vi "ResearcgStandingFrame-V2.1.vi"() -> ()   [LabVIEW 2012]
doc: "Use this template to build a simple state machine design pattern. Each state executes code and determines which state to transition to."
uses:
  controls/State.ctl
  <vilib>/DAQmx/read.llb/DAQmx Read (Analog 2D DBL NChan NSamp).vi
  <vilib>/DAQmx/create/channels.llb/DAQmx Create Channel (AI-Voltage-Basic).vi
  <vilib>/DAQmx/configure/timing.llb/DAQmx Timing (Sample Clock).vi
  <vilib>/DAQmx/create/channels.llb/DAQmx Create Channel (CO-Pulse Generation-Frequency).vi
  <vilib>/DAQmx/configure/timing.llb/DAQmx Timing (Implicit).vi
  <vilib>/DAQmx/miscellaneous.llb/DAQmx Fill In Error Info.vi
  <vilib>/Utility/file.llb/Write To Spreadsheet File (DBL).vi
panel:
  out "refnum out":refnum<file>
  in  "Tab Control":T1(tab)
  in  "?":bool
  out "Center Mass Left Force Plate":cluster{dbl[], dbl[]}(graph)={[-7.494780644696312], [-1.1979086821741642]}
  in  "Save":bool
  in  "stop":bool
  out "Newton Force Readings File Path":path=path "C:/Documents and Settings/z00323/My Documents/Standing Frame/test data/StandingFrameTEST39.dat"
  in  "Newtons":bool
  out "Voltage Readings File Path":path=path "C:/Documents and Settings/z00323/My Documents/Standing Frame/test data/StandingFrameTEST39.dat"
  out "R-FP-Z":dbl
  out "R-FP-Y":dbl
  out "R-FP-X":dbl
  out "R-LC-Z":dbl
  out "R-LC-Y":dbl
  out "R-LC-X":dbl
  out "L-LC-Z":dbl
  out "L-LC-Y":dbl
  out "L-LC-X":dbl
  out "L-FP-X":dbl
  out "L-FP-Y":dbl
  out "L-FP-Z":dbl
  out "String":string caption="Display Unit"
  out "Left Force Plate Z":dbl(slide)=0.43558763460600747 scale=0.0..250.0
  out "Right Force Plate Z":dbl(slide)=0.868584773555102 scale=0.0..250.0
  out "Center Mass Right Force Plate":cluster{dbl[], dbl[]}(graph)
  out "Right Load Cell":cluster{dbl[], dbl[]}(graph)={[0.0, -0.0006862149399022939, 0.0, 0.0], [0.0, 0.005798023167495851, 0.0, 0.0]}
  out "Right Load Cell Z":dbl(slide)=-0.000301685706272135 scale=-50.0..250.0
  out "Left Load Cell Z":dbl(slide)=-0.004073381073294343 scale=-50.0..250.0
  out "Left Load Cell":cluster{dbl[], dbl[]}(graph)={[0.0, -0.0004854170425343219, 0.0, 0.0], [0.0, -0.002818533162237429, 0.0, 0.0]}
  out "Amplitude Unit":string
  out "Right Force PLate Z":dbl(graph)
  out "Left Force Plate Z":dbl(graph)
  out "Right Load Cell Z":dbl(graph)
  out "Right Load Cell Y":dbl(graph)
  out "Right Load Cell X":dbl(graph)
  out "Left Load Cell Z":dbl(graph)
  out "Left Load Cell Y":dbl(graph)
  out "Left Load Cell X":dbl(graph)
  out "Amplitude Unit":string
  out "Loading- Clibration File Path":path
  in  "Save Calibration Results":bool
  in  "Load Previous Calibration Results":bool
  out "Saving- Clibration File Path":path
  out "Baseline Out":dbl[](array[numeric])
  out "Voltages":dbl[](array[numeric])
  in  "New Calibration":bool
  # "FP4"
  # "FP3"
  # "Left Load Cell X\n\nLeft Load Cell Y\n\nLeft Load Cell Z\n\nRight Load Cell X\n\nRight Load Cell Y\n\nRight Load Cell Z"
  # "DAQ Board Connections"
  # "Left Force Plate X1\n\nLeft Force Plate X2\n\nLeft Force Plate Y1\n\nLeft Force Plate Y2\n\nLeft Force Plate Z1\n\nLeft Force Plate Z2\n\nLeft Force Plate Z3\n\nLeft Force Plate Z4"
  # "LX\nLY\nLZ\nRX\nRY\nRZ\nLFX12\nLFX34\nLFY14\nLFY23\nLFZ1\nLFZ2\nLFZ3\nLFZ4\nRFX12\nRFX34\nRFY14\nRFY23\nRFZ1\nRFZ2\nRFZ3\nRFZ4"
  # "32\n33\n34\n35\n36\n37\n0\n1\n2\n3\n4\n5\n6\n7\n16\n17\n18\n19\n20\n21\n22\n23"
  # "Right Force Plate X1\n\nRight Force Plate X2\n\nRight Force Plate Y1\n\nRight Force Plate Y2\n\nRight Force Plate Z1\n\nRight Force Plate Z2\n\nRight Force Plate Z3\n\nRight Force Plate Z4"
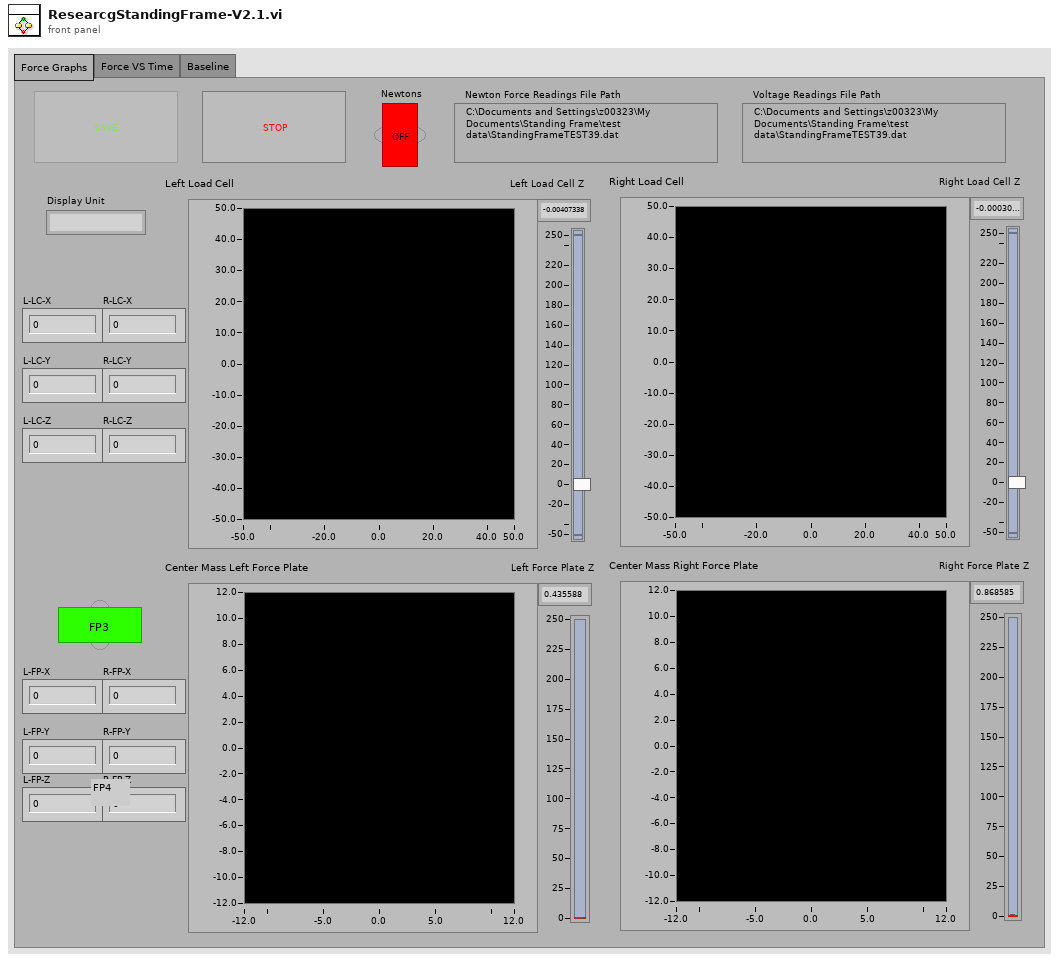
[diagram p1: front panel]
types:
  T1 = enum32{"Force Graphs", "Force VS Time", "Baseline"}
  T2 = typedef "State.ctl" = enum16{"Initialize", "Save", "Main", "Stop"}
  T3 = enum16{"open", "replace", "create", "open or create", "replace or create", "replace or create with confirmation"}
  T4 = enum8{"Enabled", "Disabled", "Disabled and Grayed Out"}
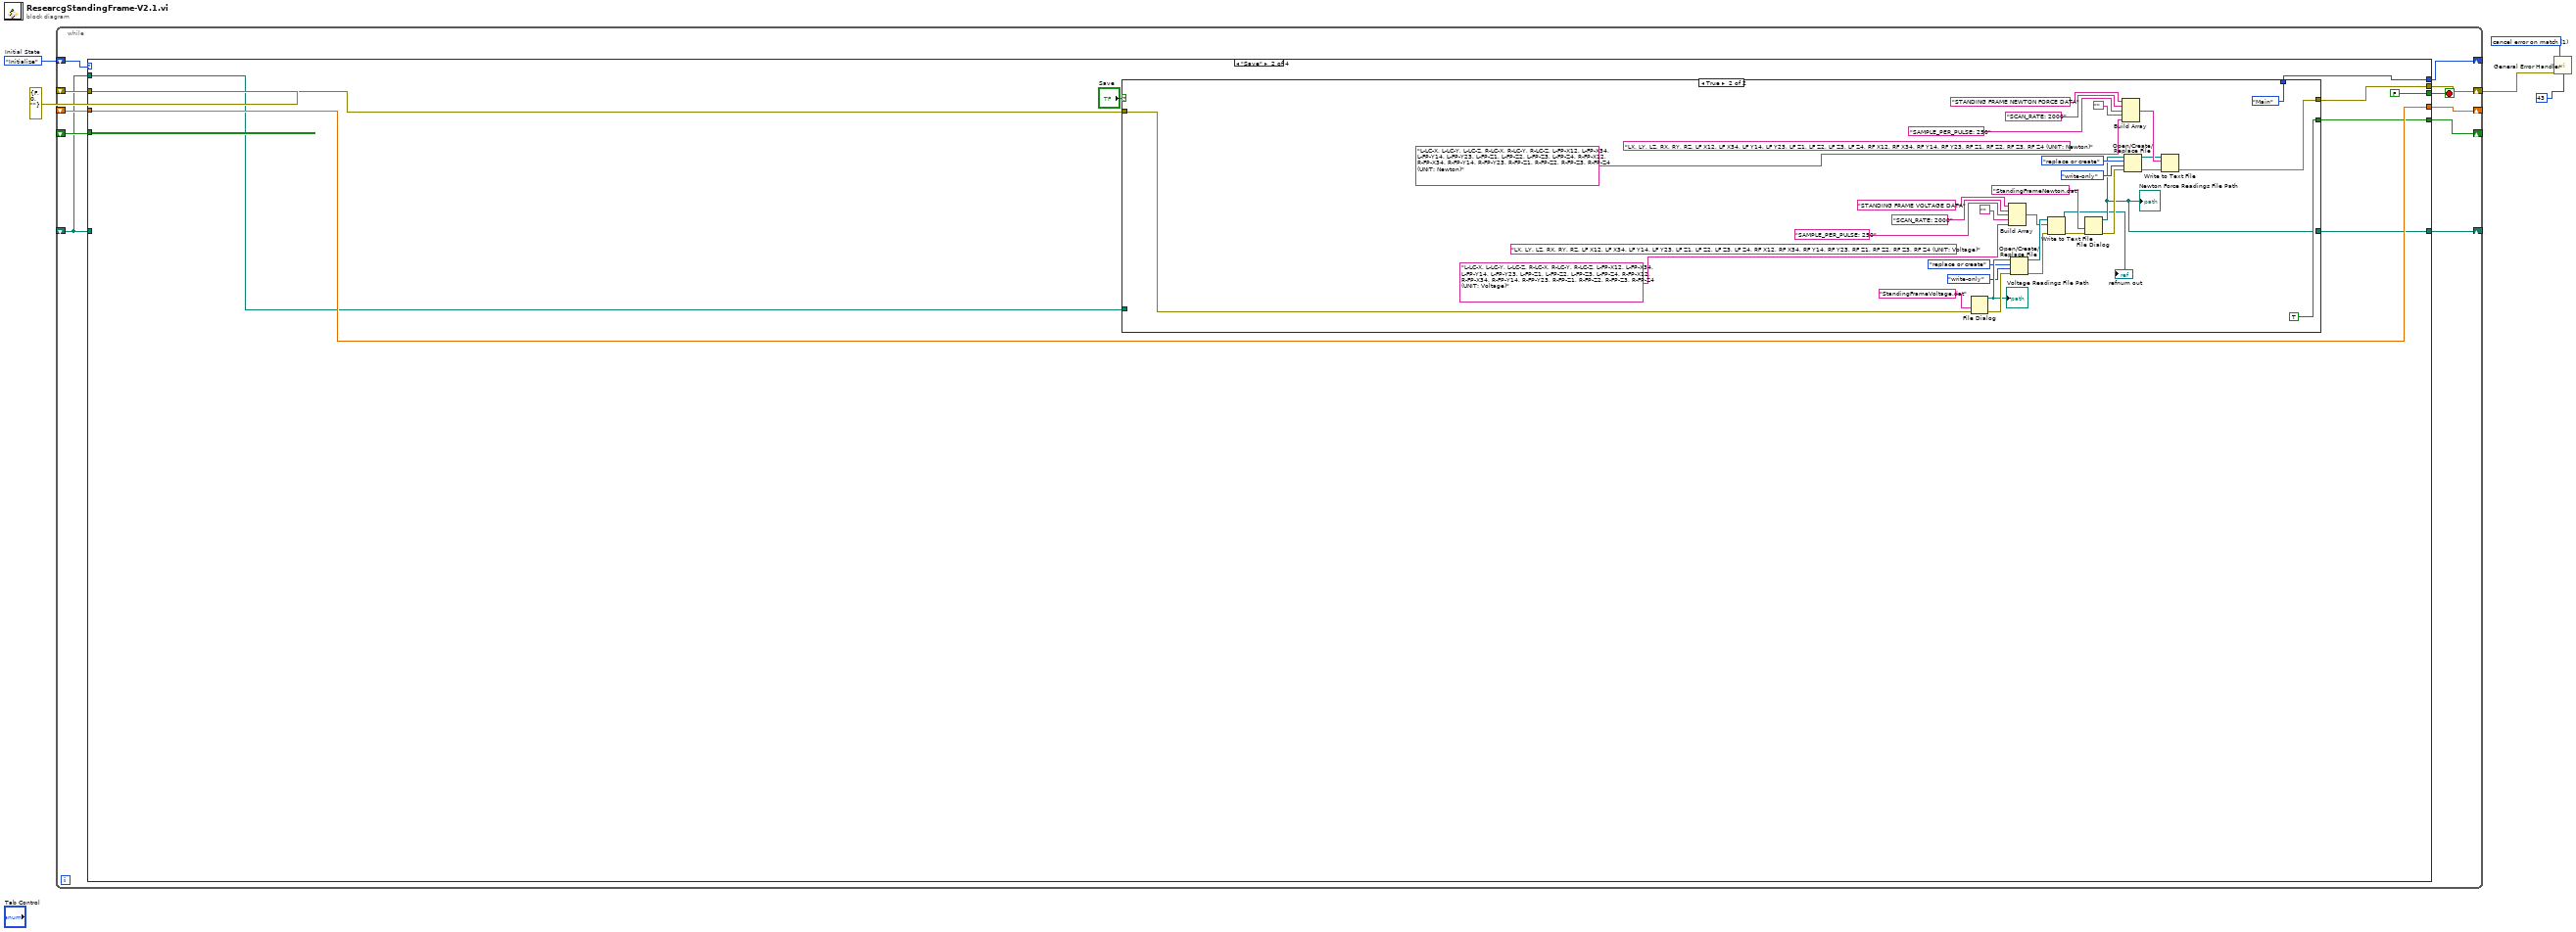
[diagram p0: block diagram]
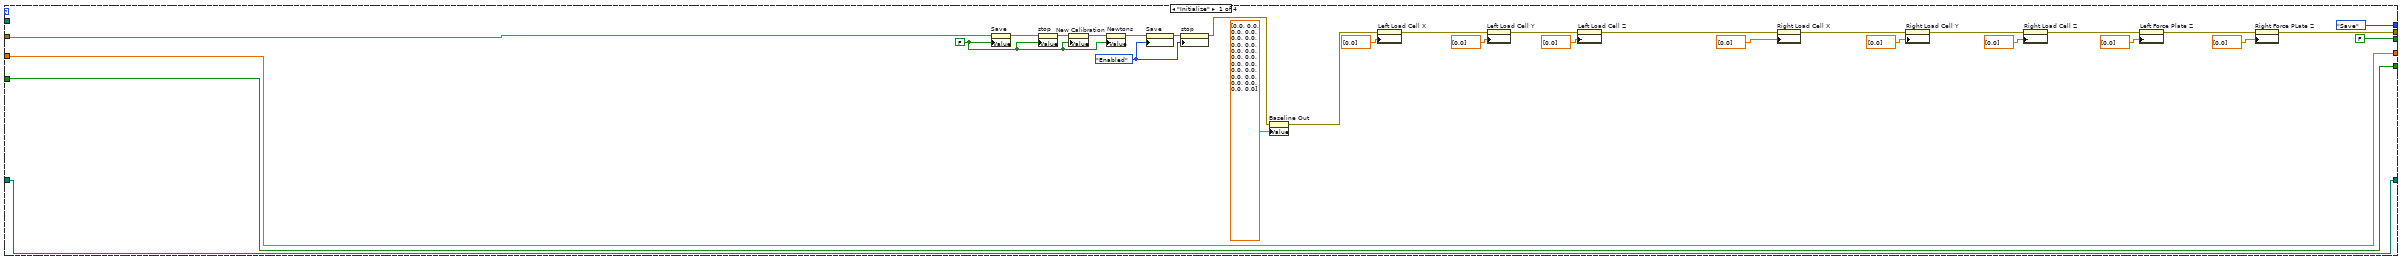
[diagram p2: hidden frame]
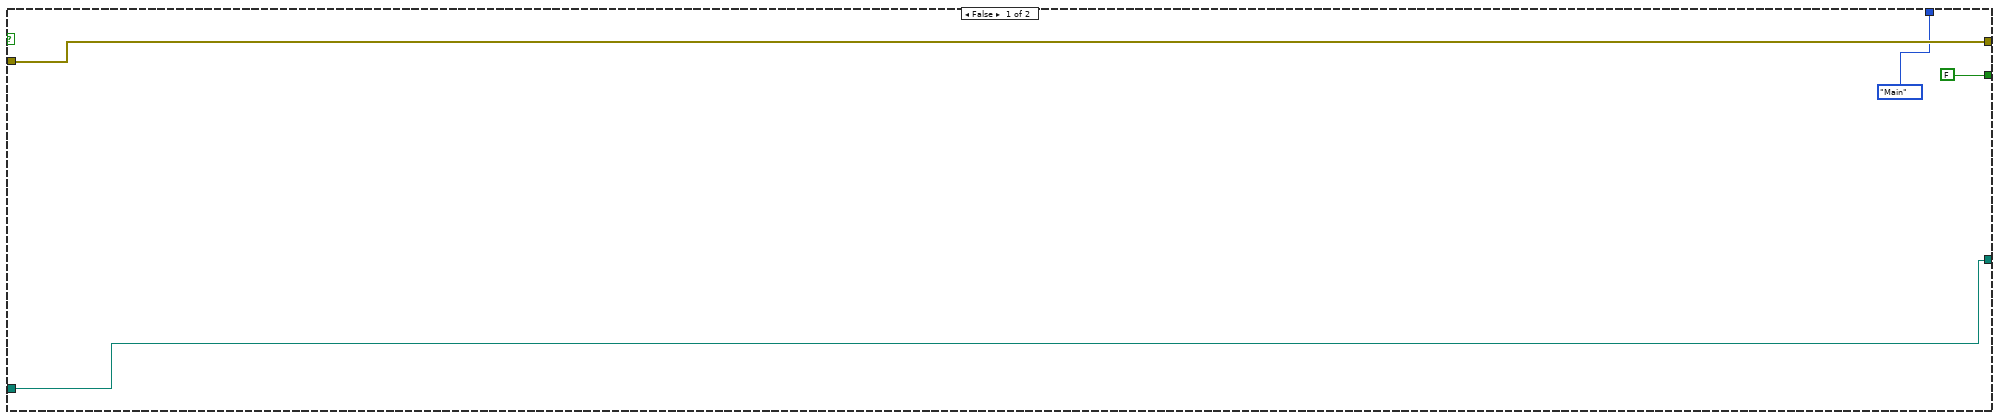
[diagram p3: hidden frame]
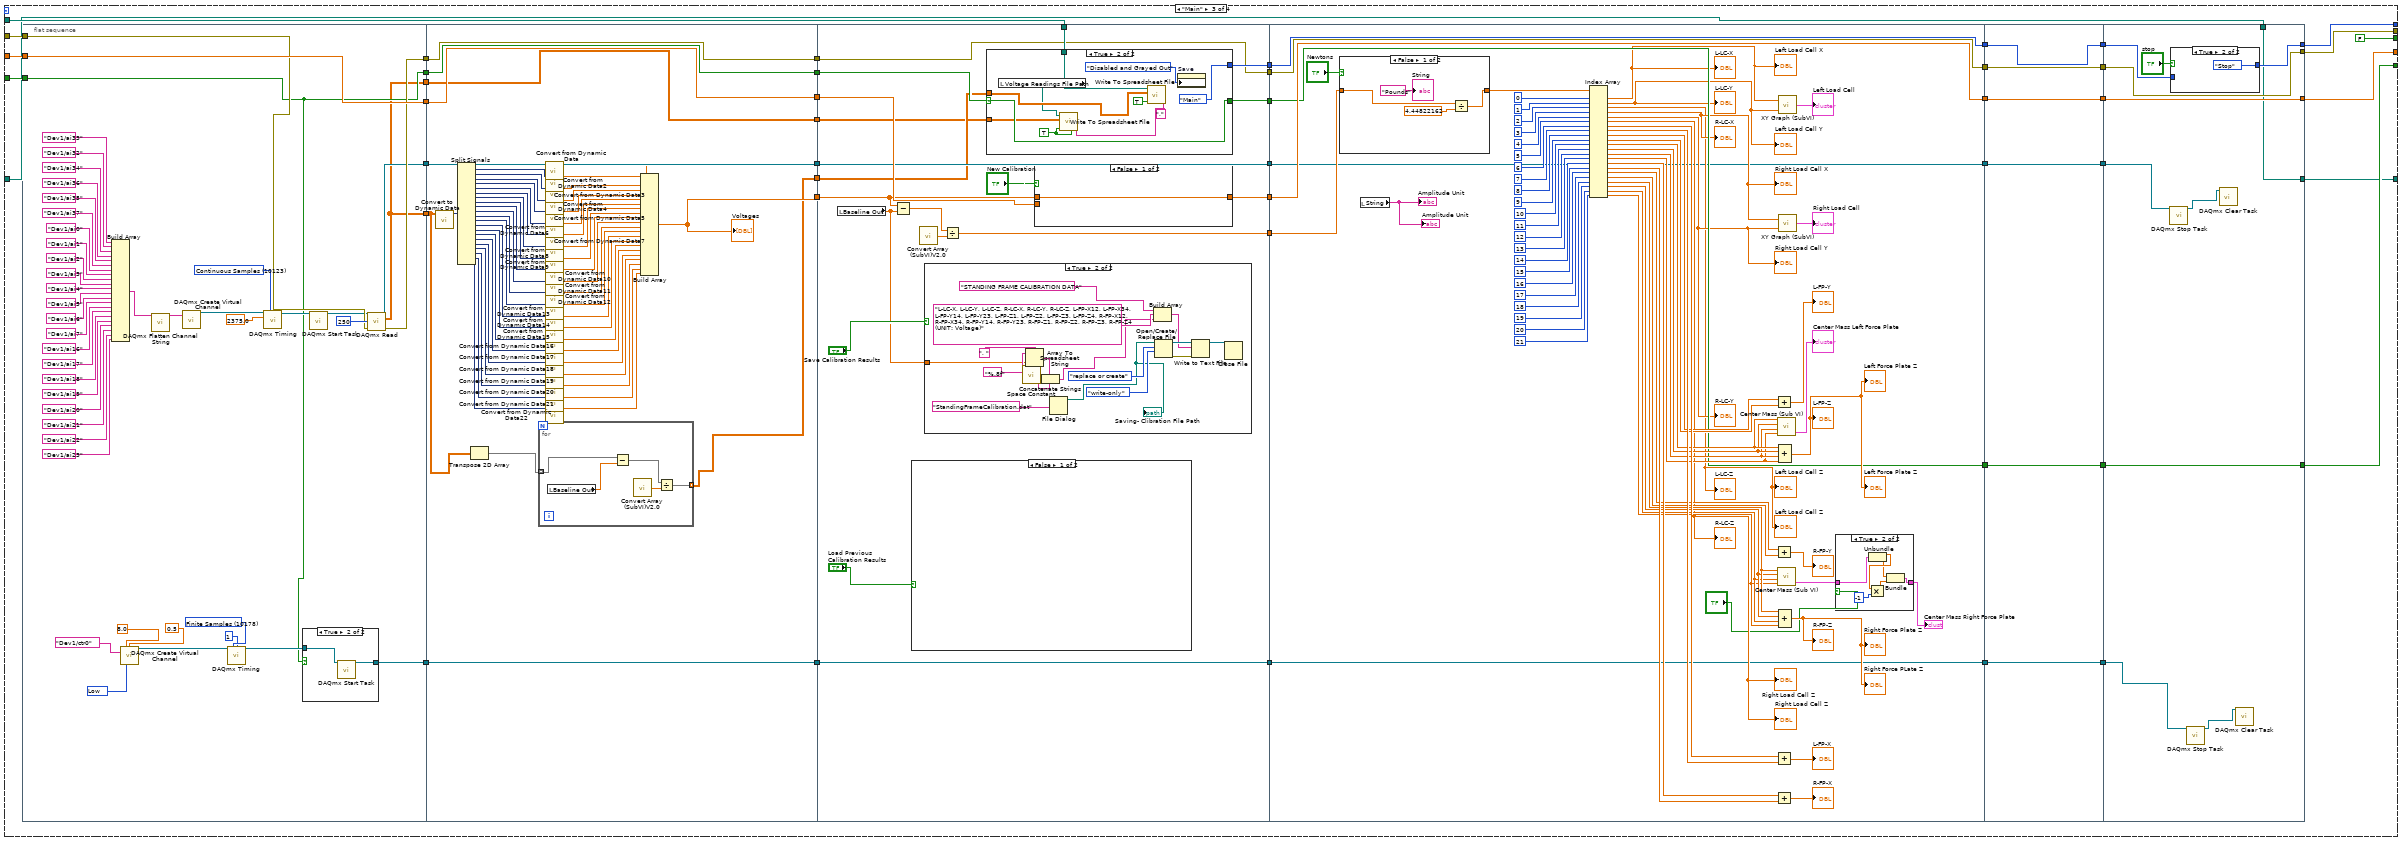
[diagram p4: hidden frame]
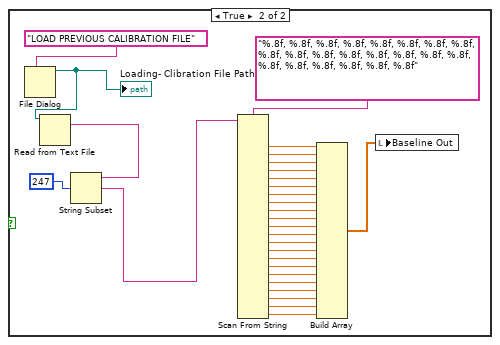
[diagram p6: hidden frame]
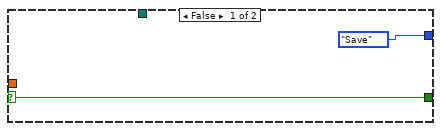
[diagram p8: hidden frame]
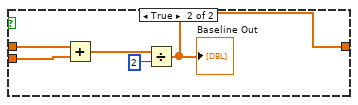
[diagram p9: hidden frame]
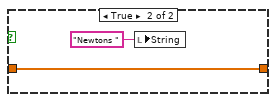
[diagram p11: hidden frame]
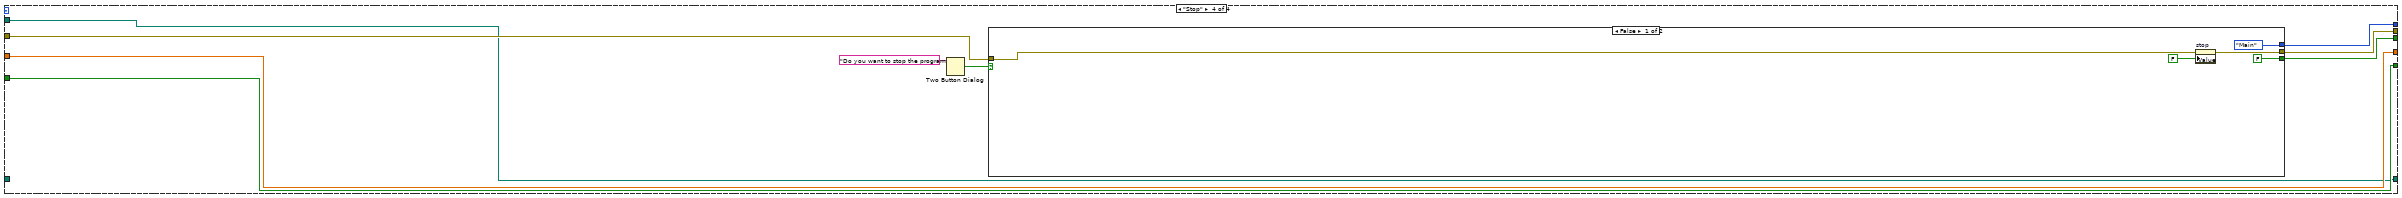
[diagram p13: hidden frame]
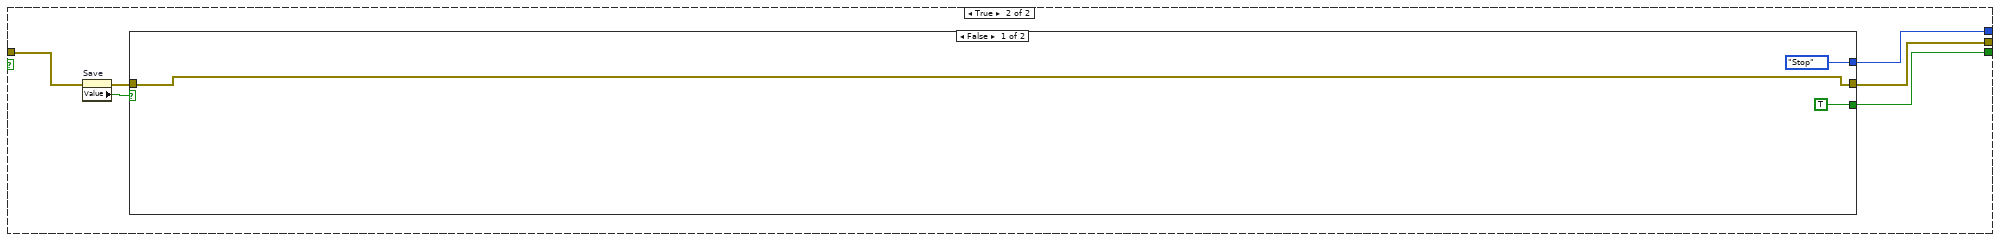
[diagram p14: hidden frame]
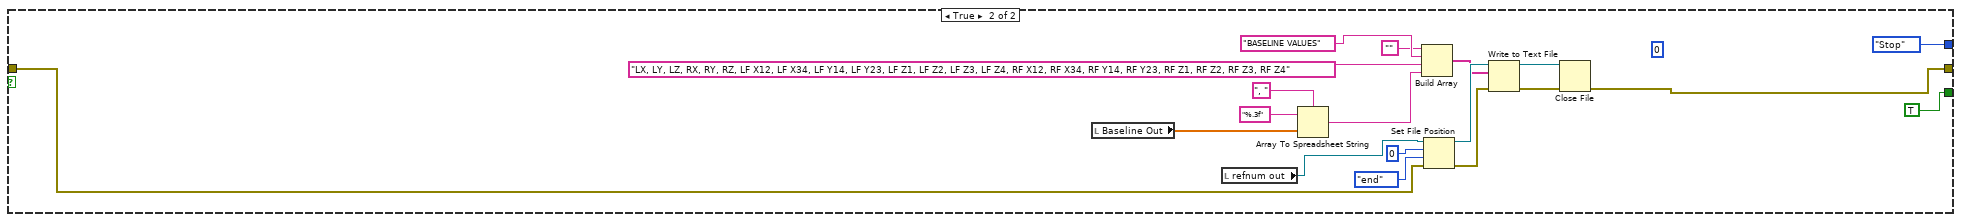
[diagram p15: hidden frame]
diagram:
  w1 = 1 items=["no exception", "cancel error on match", "set error on match"] ("[exception action] (none:0)")
  w5 = State."Initialize"  # Initial State
  n1 = while {
    shift-right: [w16] -> _
    shift-left: w5 -> [w6]
    shift-right: [w13] -> w3
    shift-left: errorcluster {"status"=FALSE, "code"=0, "source"=""} ("error out") -> [w15]
    shift-right: [w11] -> _
    shift-left: _ -> [w12]
    shift-right: [w10] -> _
    shift-left: _ -> [w9]
    shift-right: [w8] -> _
    shift-left: _ -> [w7]
    stop <- w14 stop-if-true
    n2 = case shown="\"Save\"" w6 {
      tunnel: [State."Save" ("Next State") w51 w137 w433] -> w16
      tunnel: [FALSE ("T button?") FALSE FALSE ("T button?") w432] -> w14
      tunnel: w15 -> [w43 w56 w138 w431]
      tunnel: [w20 w55 w127 w430] -> w13
      tunnel: w12 -> [w42 w53 w125 w429]
      tunnel: [w42 w53 w121 w429] -> w11
      tunnel: [w18 w52 w118 w428] -> w10
      tunnel: w9 -> [w18 _ w119 w428]
      tunnel: [w17 w50 w94 w427] -> w8
      tunnel: w7 -> [_ w49 w96 w427]
      tunnel: w7 -> [w17 _ w95 _]
      frame "Initialize" {
        w37 = FALSE ("Begin")
        w46 = T4."Enabled" ("Disabled")
        n3 = property on="Save" class="Bool (strict)"(error in=w43, "Value"=w37) -> (error out=w45:errorcluster)  [unwired: 1 in, 1 out]
        n4 = property on="stop" class="Bool (strict)"(error in=w45, "Value"=w37) -> (error out=w41:errorcluster)  [unwired: 1 in, 1 out]
        n5 = property on="New Calibration" class="Bool (strict)"(error in=w41, "Value"=w37) -> (error out=w39:errorcluster)  [unwired: 1 in, 1 out]
        n6 = property on="Newtons" class="Bool (strict)"(error in=w39, "Value"=w37) -> (error out=w38:errorcluster)  [unwired: 1 in, 1 out]
        n7 = property on="Save" class="Bool (strict)"(error in=w38, "DisabledEnum"=w46) -> (error out=w44:errorcluster)  [unwired: 1 in, 1 out]
        n8 = property on="stop" class="Bool (strict)"(error in=w44, "DisabledEnum"=w46) -> (error out=w19:errorcluster)  [unwired: 1 in, 1 out]
        n9 = property on="Baseline Out" class="Arr (strict)"(error in=w19, "Value"=dbl[] [0.0, 0.0, 0.0, 0.0, 0.0, 0.0, 0.0, 0.0, 0.0, 0.0, 0.0, 0.0, 0.0, 0.0, 0.0, 0.0, 0.0, 0.0, 0.0, 0.0, 0.0, 0.0] ("Baseline Out")) -> (error out=w28:errorcluster)  [unwired: 1 in, 1 out]
        n10 = property on="Left Load Cell X" class="WFChart (strict)"(error in=w28, "History Data"=dbl[] [0.0]) -> (error out=w27:errorcluster)  [unwired: 1 in, 1 out]
        n11 = property on="Left Load Cell Y" class="WFChart (strict)"(error in=w27, "History Data"=dbl[] [0.0]) -> (error out=w26:errorcluster)  [unwired: 1 in, 1 out]
        n12 = property on="Left Load Cell Z" class="WFChart (strict)"(error in=w26, "History Data"=dbl[] [0.0]) -> (error out=w25:errorcluster)  [unwired: 1 in, 1 out]
        n13 = property on="Right Load Cell X" class="WFChart (strict)"(error in=w25, "History Data"=dbl[] [0.0]) -> (error out=w24:errorcluster)  [unwired: 1 in, 1 out]
        n14 = property on="Right Load Cell Y" class="WFChart (strict)"(error in=w24, "History Data"=dbl[] [0.0]) -> (error out=w23:errorcluster)  [unwired: 1 in, 1 out]
        n15 = property on="Right Load Cell Z" class="WFChart (strict)"(error in=w23, "History Data"=dbl[] [0.0]) -> (error out=w22:errorcluster)  [unwired: 1 in, 1 out]
        n16 = property on="Left Force Plate Z" class="WFChart (strict)"(error in=w22, "History Data"=dbl[] [0.0]) -> (error out=w21:errorcluster)  [unwired: 1 in, 1 out]
        n17 = property on="Right Force PLate Z" class="WFChart (strict)"(error in=w21, "History Data"=dbl[] [0.0]) -> (error out=w20:errorcluster)  [unwired: 1 in, 1 out]
      }
      frame "Save" {
        n18 = case shown="True" "Save" {
          tunnel: w56 -> [w61 w75]
          tunnel: [w61 w89] -> w55
          tunnel: [FALSE TRUE] -> w52
          tunnel: [State."Main" ("Next State") State."Main" ("Next State")] -> w51
          tunnel: [w58 w63] -> w50
          tunnel: w49 -> [w58 _]
          frame False {
          }
          frame True {
            (unwired) "LX, LY, LZ, RX, RY, RZ, LF X12, LF X34, LF Y14, LF Y23, LF Z1, LF Z2, LF Z3, LF Z4, RF X12, RF X34, RF Y14, RF Y23, RF Z1, RF Z2, RF Z3, RF Z4 (UNIT: Voltage)"
            (unwired) "LX, LY, LZ, RX, RY, RZ, LF X12, LF X34, LF Y14, LF Y23, LF Z1, LF Z2, LF Z3, LF Z4, RF X12, RF X34, RF Y14, RF Y23, RF Z1, RF Z2, RF Z3, RF Z4 (UNIT: Newton)"
            n19 = File Dialog(8:w75, 9:"StandingFrameVoltage.dat" ("default name")) -> (0:w83:errorcluster, 3:w81:path)  [unwired: 1 in, 6 out]
            "Voltage Readings File Path" <- w81
            n20 = Build Array("STANDING FRAME VOLTAGE DATA", "SCAN_RATE: 2000", "SAMPLE_PER_PULSE: 250", "", "L-LC-X, L-LC-Y, L-LC-Z, R-LC-X, R-LC-Y, R-LC-Z, L-FP-X12, L-FP-X34, L-FP-Y14, L-FP-Y23, L-FP-Z1, L-FP-Z2, L-FP-Z3, L-FP-Z4, R-FP-X12, R-FP-X34, R-FP-Y14, R-FP-Y23, R-FP-Z1, R-FP-Z2, R-FP-Z3, R-FP-Z4 (UNIT: Voltage)") -> (w79:string[])
            n21 = Open/Create/Replace File(file path (use dialog)=w81, error in=w83, operation (0:open)=T3."replace or create", access (0:read/write)=enum16{"read/write", "read-only", "write-only"}."write-only") -> (refnum out=w80:refnum<file>, error out=w84:errorcluster)  [unwired: 3 out]
            n22 = Write to Text File(file (use dialog)=w80, text=w79, error in=w84) -> (refnum out=→"refnum out":refnum<file>, error out=w74:errorcluster)  [unwired: 1 in, 1 out]
            n23 = File Dialog(8:w74, 9:"StandingFrameNewton.dat" ("default name")) -> (0:w86:errorcluster, 3:w63:path)  [unwired: 1 in, 6 out]
            "Newton Force Readings File Path" <- w63
            n24 = Build Array("STANDING FRAME NEWTON FORCE DATA", "SCAN_RATE: 2000", "SAMPLE_PER_PULSE: 250", "", "L-LC-X, L-LC-Y, L-LC-Z, R-LC-X, R-LC-Y, R-LC-Z, L-FP-X12, L-FP-X34, L-FP-Y14, L-FP-Y23, L-FP-Z1, L-FP-Z2, L-FP-Z3, L-FP-Z4, R-FP-X12, R-FP-X34, R-FP-Y14, R-FP-Y23, R-FP-Z1, R-FP-Z2, R-FP-Z3, R-FP-Z4 (UNIT: Newton)") -> (w90:string[])
            n25 = Open/Create/Replace File(file path (use dialog)=w63, error in=w86, operation (0:open)=T3."replace or create", access (0:read/write)=enum16{"read/write", "read-only", "write-only"}."write-only") -> (refnum out=w88:refnum<file>, error out=w85:errorcluster)  [unwired: 3 out]
            n26 = Write to Text File(file (use dialog)=w88, text=w90, error in=w85) -> (error out=w89:errorcluster)  [unwired: 1 in, 2 out]
          }
        }
      }
      frame "Main" {
        n27 = flat-sequence {
          tunnel: w138 -> [w169]
          tunnel: [w168] -> w135
          tunnel: [w183] -> w126
          tunnel: w125 -> [w183]
          tunnel: [w142] -> w120
          tunnel: w119 -> [w142]
          tunnel: [w167] -> w106
          tunnel: [w139] -> w105
          tunnel: [w143] -> w100
          tunnel: [w139] -> w97
          tunnel: [w241] -> w114
          tunnel: [w240] -> w113
          tunnel: [w239] -> w112
          tunnel: [w238] -> w111
          tunnel: [w237] -> w107
          tunnel: [w236] -> w101
          tunnel: w100 -> [w236]
          tunnel: w105 -> [w188]
          tunnel: w106 -> [w237]
          tunnel: w120 -> [w238]
          tunnel: w126 -> [w240]
          tunnel: w135 -> [w241]
          tunnel: [w195] -> w99
          tunnel: [w196] -> w98
          tunnel: w97 -> [w196]
          tunnel: [w264] -> w134
          tunnel: w114 -> [w247]
          tunnel: [w247] -> w133
          tunnel: [w251] -> w132
          tunnel: w113 -> [w263]
          tunnel: w112 -> [w262]
          tunnel: [w261] -> w124
          tunnel: w111 -> [w258]
          tunnel: [w257] -> w115
          tunnel: [w253] -> w108
          tunnel: w107 -> [w253]
          tunnel: [w252] -> w102
          tunnel: w101 -> [w252]
          tunnel: w99 -> [w250]
          tunnel: w98 -> [w249]
          tunnel: w96 -> [w248]
          tunnel: w134 -> [w394]
          tunnel: [w394] -> w131
          tunnel: w133 -> [w343]
          tunnel: w132 -> [w392]
          tunnel: [w343] -> w129
          tunnel: w124 -> [w358]
          tunnel: [w358] -> w123
          tunnel: [w344] -> w116
          tunnel: w115 -> [w344]
          tunnel: [w333] -> w109
          tunnel: w108 -> [w333]
          tunnel: [w332] -> w103
          tunnel: w102 -> [w332]
          tunnel: w131 -> [w413]
          tunnel: [w413] -> w130
          tunnel: w129 -> [w412]
          tunnel: [w412] -> w128
          tunnel: w123 -> [w411]
          tunnel: [w411] -> w122
          tunnel: [w410] -> w117
          tunnel: w116 -> [w410]
          tunnel: [w409] -> w110
          tunnel: w109 -> [w409]
          tunnel: [w408] -> w104
          tunnel: w103 -> [w408]
          tunnel: [w424] -> w137
          tunnel: w130 -> [w422]
          tunnel: w128 -> [w421]
          tunnel: [w421] -> w127
          tunnel: w122 -> [w420]
          tunnel: [w420] -> w121
          tunnel: [w419] -> w118
          tunnel: w117 -> [w419]
          tunnel: w110 -> [w418]
          tunnel: w104 -> [w415]
          tunnel: w95 -> [w414]
          tunnel: [w414] -> w94
          frame #0 {
            w173 = 10178 items=["Finite Samples"=10178, "Continuous Samples"=10123, "Hardware Timed Single Point"=12522] ("sample mode")
            w175 = 10214 items=["High"=10192, "Low"=10214] ("idle state")
            w180 = 10123 items=["Finite Samples"=10178, "Continuous Samples"=10123, "Hardware Timed Single Point"=12522] ("Sample Mode:")
            n28 = Build Array("Dev1/ai33" ("string"), "Dev1/ai32" ("string"), "Dev1/ai34" ("string"), "Dev1/ai36" ("string"), "Dev1/ai35" ("string"), "Dev1/ai37" ("string"), "Dev1/ai0" ("string"), "Dev1/ai1" ("string"), "Dev1/ai2" ("string"), "Dev1/ai3" ("string"), "Dev1/ai4" ("string"), "Dev1/ai5" ("string"), "Dev1/ai6" ("string"), "Dev1/ai7" ("string"), "Dev1/ai16" ("string"), "Dev1/ai17" ("string"), "Dev1/ai18" ("string"), "Dev1/ai19" ("string"), "Dev1/ai20" ("string"), "Dev1/ai21" ("string"), "Dev1/ai22" ("string"), "Dev1/ai23" ("string")) -> (w140:string[])
            n29 = call-poly <vilib>:"DAQmx Create Virtual Channel.vi"("frequency"=8.0, "duty cycle"=0.5, "counter"=tag "Dev1/ctr0" ("Pulse Output Channel"), "idle state"=w175) -> ("task out"=w174:refnum<k21>)  [unwired: 10 in, 1 out]
            n30 = call <vilib>:"DAQmx Flatten Channel String.vi"("names in"=w140) -> ("names out"=w182:string)  [unwired: 13 in, 1 out]
            n31 = call-poly <vilib>:"DAQmx Create Virtual Channel.vi"("physical channels"=w182) -> ("task out"=w181:refnum<k21>)  [unwired: 13 in, 1 out]
            n32 = call-poly <vilib>:"DAQmx Timing.vi"("task/channels in"=w174, "sample mode"=w173, "samples per channel"=1) -> ("task out"=w144:refnum<k21>)  [unwired: 11 in, 1 out]
            n33 = call-poly <vilib>:"DAQmx Timing.vi"("task/channels in"=w181, "sample mode"=w180, "rate"=sgl 2375.0 ("Scan Rate:")) -> ("task out"=w171:refnum<k21>)  [unwired: 11 in, 1 out]
            n34 = case shown="True" w142 {
              tunnel: w144 -> [w184 w186]
              tunnel: [w184 w185] -> w143
              frame False {
              }
              frame True {
                n35 = call <vilib>:"DAQmx Start Task.vi"("task/channels in"=w186) -> ("task out"=w185:refnum<k21>)  [unwired: 13 in, 1 out]
              }
            }
            n36 = call <vilib>:"DAQmx Start Task.vi"("task/channels in"=w171) -> ("task out"=w141:refnum<k21>)  [unwired: 13 in, 1 out]
            n37 = call-poly <vilib>:"DAQmx Read.vi"("task/channels in"=w141, "number of samples per channel"=250, "error in"=w169) -> ("task out"=w167:refnum<k21>, "data"=w139:dbl[][], "error out"=w168:errorcluster)  [unwired: 10 in]
          }
          frame #1 {
            n38 = call "Convert to Dynamic Data"("2D Array"=w188) -> ("Dynamic Data Type"=w197:dynamicdata)  [unwired: 3 in]
            n39 = Split Signals(w197) -> (w235:dynamicdata, w234:dynamicdata, w233:dynamicdata, w232:dynamicdata, w231:dynamicdata, w230:dynamicdata, w229:dynamicdata, w228:dynamicdata, w227:dynamicdata, w226:dynamicdata, w225:dynamicdata, w224:dynamicdata, w223:dynamicdata, w222:dynamicdata, w221:dynamicdata, w220:dynamicdata, w219:dynamicdata, w218:dynamicdata, w217:dynamicdata, w216:dynamicdata, w215:dynamicdata, w214:dynamicdata)  [unwired: 22 in]
            n40 = Transpose 2D Array(2D array=w188) -> (transposed array=w189:dbl[][])
            n41 = for {
              tunnel: w189 -> [w242] mode=indexing
              tunnel: [w243] -> w195 mode=indexing
              n42 = local read "Baseline Out"() -> (w246:dbl[])
              n43 = Subtract(x=w242, y=w246) -> (x-y=w245:dbl[])
              n44 = call "Convert Array  (SubVI)V2.0.vi"() -> ("Conversion Array"=w244:dbl[])  [unwired: 1 in]
              n45 = Divide(x=w245, y=w244) -> (x/y=w243:dbl[])
            }
            n46 = call "Convert from Dynamic Data"("Dynamic Data Type"=w235) -> ("Scalar"=w193:dbl)  [unwired: 3 in]
            n47 = call "Convert from Dynamic Data2"("Dynamic Data Type"=w234) -> ("Scalar"=w194:dbl)  [unwired: 3 in]
            n48 = call "Convert from Dynamic Data3"("Dynamic Data Type"=w233) -> ("Scalar"=w187:dbl)  [unwired: 3 in]
            n49 = call "Convert from Dynamic Data4"("Dynamic Data Type"=w232) -> ("Scalar"=w192:dbl)  [unwired: 3 in]
            n50 = call "Convert from Dynamic Data5"("Dynamic Data Type"=w231) -> ("Scalar"=w191:dbl)  [unwired: 3 in]
            n51 = call "Convert from Dynamic Data6"("Dynamic Data Type"=w230) -> ("Scalar"=w190:dbl)  [unwired: 3 in]
            n52 = call "Convert from Dynamic Data7"("Dynamic Data Type"=w229) -> ("Scalar"=w202:dbl)  [unwired: 3 in]
            n53 = call "Convert from Dynamic Data8"("Dynamic Data Type"=w228) -> ("Scalar"=w203:dbl)  [unwired: 3 in]
            n54 = call "Convert from Dynamic Data9"("Dynamic Data Type"=w227) -> ("Scalar"=w204:dbl)  [unwired: 3 in]
            n55 = call "Convert from Dynamic Data10"("Dynamic Data Type"=w226) -> ("Scalar"=w205:dbl)  [unwired: 3 in]
            n56 = call "Convert from Dynamic Data11"("Dynamic Data Type"=w225) -> ("Scalar"=w201:dbl)  [unwired: 3 in]
            n57 = call "Convert from Dynamic Data12"("Dynamic Data Type"=w224) -> ("Scalar"=w200:dbl)  [unwired: 3 in]
            n58 = call "Convert from Dynamic Data13"("Dynamic Data Type"=w223) -> ("Scalar"=w206:dbl)  [unwired: 3 in]
            n59 = call "Convert from Dynamic Data14"("Dynamic Data Type"=w222) -> ("Scalar"=w199:dbl)  [unwired: 3 in]
            n60 = call "Convert from Dynamic Data15"("Dynamic Data Type"=w221) -> ("Scalar"=w198:dbl)  [unwired: 3 in]
            n61 = call "Convert from Dynamic Data16"("Dynamic Data Type"=w220) -> ("Scalar"=w207:dbl)  [unwired: 3 in]
            n62 = call "Convert from Dynamic Data17"("Dynamic Data Type"=w219) -> ("Scalar"=w208:dbl)  [unwired: 3 in]
            n63 = call "Convert from Dynamic Data18"("Dynamic Data Type"=w218) -> ("Scalar"=w209:dbl)  [unwired: 3 in]
            n64 = call "Convert from Dynamic Data19"("Dynamic Data Type"=w217) -> ("Scalar"=w210:dbl)  [unwired: 3 in]
            n65 = call "Convert from Dynamic Data20"("Dynamic Data Type"=w216) -> ("Scalar"=w211:dbl)  [unwired: 3 in]
            n66 = call "Convert from Dynamic Data21"("Dynamic Data Type"=w215) -> ("Scalar"=w212:dbl)  [unwired: 3 in]
            n67 = call "Convert from Dynamic Data22"("Dynamic Data Type"=w214) -> ("Scalar"=w213:dbl)  [unwired: 3 in]
            n68 = Build Array(w193, w194, w187, w192, w191, w190, w202, w203, w204, w205, w201, w200, w206, w199, w198, w207, w208, w209, w210, w211, w212, w213) -> (w239:dbl[])
            "Voltages" <- w239
          }
          frame #2 {
            n69 = local read "Baseline Out"() -> (w255:dbl[])
            n70 = Subtract(x=w262, y=w255) -> (x-y=w260:dbl[])
            n71 = case shown="False" "Load Previous Calibration Results" {
              frame False {
              }
              frame True {
                n72 = File Dialog(7:"LOAD PREVIOUS CALIBRATION FILE") -> (3:w266:path)  [unwired: 2 in, 7 out]
                "Loading- Clibration File Path" <- w266
                n73 = Read from Text File(file (use dialog)=w266) -> (text=w272:string)  [unwired: 3 in, 3 out]
                n74 = String Subset(string=w272, offset (0)=247) -> (substring=w270:string)  [unwired: 1 in]
                n75 = Scan From String(format string="%.8f, %.8f, %.8f, %.8f, %.8f, %.8f, %.8f, %.8f, %.8f, %.8f, %.8f, %.8f, %.8f, %.8f, %.8f, %.8f, %.8f, %.8f, %.8f, %.8f, %.8f, %.8f", input string=w270) -> (output 1=w294:dbl, output 2=w293:dbl, output 3=w292:dbl, output 4=w291:dbl, output 5=w290:dbl, output 6=w289:dbl, output 7=w288:dbl, output 8=w287:dbl, output 9=w286:dbl, output 10=w285:dbl, output 11=w284:dbl, output 12=w283:dbl, output 13=w282:dbl, output 14=w281:dbl, output 15=w280:dbl, output 16=w279:dbl, output 17=w278:dbl, output 18=w277:dbl, output 19=w276:dbl, output 20=w275:dbl, output 21=w274:dbl, output 22=w273:dbl)  [unwired: 24 in, 3 out]
                n76 = Build Array(w294, w293, w292, w291, w290, w289, w288, w287, w286, w285, w284, w283, w282, w281, w280, w279, w278, w277, w276, w275, w274, w273) -> (w269:dbl[])
                n77 = local write "Baseline Out"(w269) -> ()
              }
            }
            n78 = call "Convert Array  (SubVI)V2.0.vi"() -> ("Conversion Array"=w259:dbl[])  [unwired: 1 in]
            n79 = case shown="True" "Save Calibration Results" {
              tunnel: w255 -> [_ w303]
              frame False {
              }
              frame True {
                n80 = call <vilib>:"Space Constant.vi"() -> ("String"=w298:string)
                n81 = Array To Spreadsheet String(delimiter (Tab)=", ", array=w303, 3:"%.8f") -> (spreadsheet string=w297:string)
                n82 = Concatenate Strings(w298, w297) -> (w296:string)
                n83 = File Dialog(9:"StandingFrameCalibration.dat" ("default name")) -> (3:w295:path)  [unwired: 2 in, 7 out]
                "Saving- Clibration File Path" <- w295
                n84 = Build Array("STANDING FRAME CALIBRATION DATA", "L-LC-X, L-LC-Y, L-LC-Z, R-LC-X, R-LC-Y, R-LC-Z, L-FP-X12, L-FP-X34, L-FP-Y14, L-FP-Y23, L-FP-Z1, L-FP-Z2, L-FP-Z3, L-FP-Z4, R-FP-X12, R-FP-X34, R-FP-Y14, R-FP-Y23, R-FP-Z1, R-FP-Z2, R-FP-Z3, R-FP-Z4 (UNIT: Voltage)", w296) -> (w308:string[])
                n85 = Open/Create/Replace File(file path (use dialog)=w295, operation (0:open)=T3."replace or create", access (0:read/write)=enum16{"read/write", "read-only", "write-only"}."write-only") -> (refnum out=w309:refnum<file>, error out=w310:errorcluster)  [unwired: 1 in, 3 out]
                n86 = Write to Text File(file (use dialog)=w309, text=w308, error in=w310) -> (refnum out=w301:refnum<file>)  [unwired: 1 in, 2 out]
                n87 = Close File(refnum=w301) -> ()  [unwired: 1 in, 2 out]
              }
            }
            n88 = Divide(x=w260, y=w259) -> (x/y=w251:dbl[])
            n89 = case shown="True" w258 {
              selector: w258 -> [w311 w320]
              tunnel: [State."Save" ("(Value Not Used)") State."Main" ("(Value Not Used)")] -> w264
              tunnel: w250 -> [_ w319]
              tunnel: [w311 w320] -> w257
              tunnel: w249 -> [_ w316]
              tunnel: w248 -> [_ w317]
              frame False {
              }
              frame True {
                w315 = TRUE ("append to file? (new file:F)")
                w314 = "," ("delimiter (\\t)")
                n90 = local read "Voltage Readings File Path"() -> (w313:path)
                n91 = call-poly <vilib>:"Write To Spreadsheet File.vi"("delimiter (\\t)"=w314, "transpose? (no:F)"=w315, "append to file? (new file:F)"=w315, "2D data"=w316, "file path (dialog if empty)"=w313) -> ()  [unwired: 3 in, 1 out]
                n92 = call-poly <vilib>:"Write To Spreadsheet File.vi"("delimiter (\\t)"=w314, "append to file? (new file:F)"=TRUE, "2D data"=w319, "file path (dialog if empty)"=w317) -> ()  [unwired: 4 in, 1 out]
                n93 = property on="Save" class="Bool (strict)"("DisabledEnum"=T4."Disabled and Grayed Out" ("Disabled")) -> ()  [unwired: 2 in, 2 out]
              }
            }
            n94 = case shown="False" "New Calibration" {
              tunnel: w263 -> [_ w324]
              tunnel: w262 -> [w323 w326]
              tunnel: [w323 w325] -> w261
              frame False {
              }
              frame True {
                n95 = Add(x=w326, y=w324) -> (x+y=w328:dbl[])
                n96 = Divide(x=w328, y=2) -> (x/y=w325:dbl[])
                "Baseline Out" <- w325
              }
            }
          }
          frame #3 {
            n97 = case shown="False" "Newtons" {
              tunnel: w392 -> [w404 w406]
              tunnel: [w403 w406] -> w391
              frame False {
                n98 = Divide(x=w404, y=4.44822162) -> (x/y=w403:dbl[])
                "String" <- "Pounds" ("String")
              }
              frame True {
                n99 = local write "String"("Newtons " ("String")) -> ()
              }
            }
            n100 = local read "String"() -> (→"Amplitude Unit" →"Amplitude Unit":string)
            n101 = Index Array(array=w391, index #1=0 ("index (row)"), index #2=1 ("index (row)"), index #3=2 ("index (row)"), index #4=3 ("index (row)"), index #5=4 ("index (row)"), index #6=5 ("index (row)"), index #7=6 ("index (row)"), index #8=7 ("index (row)"), index #9=8 ("index (row)"), index #10=9 ("index (row)"), index #11=10 ("index (row)"), index #12=11 ("index (row)"), index #13=12 ("index (row)"), index #14=13 ("index (row)"), index #15=14 ("index (row)"), index #16=15 ("index (row)"), index #17=16 ("index (row)"), index #18=17 ("index (row)"), index #19=18 ("index (row)"), index #20=19 ("index (row)"), index #21=20 ("index (row)"), index #22=21 ("index (row)")) -> (element #1=w337:dbl, element #2=w338:dbl, element #3=→"L-LC-Z" →"Left Load Cell Z" →"Left Load Cell Z":dbl, element #4=w339:dbl, element #5=w340:dbl, element #6=→"R-LC-Z" →"Right Load Cell Z" →"Right Load Cell Z":dbl, element #7=w368:dbl, element #8=w367:dbl, element #9=w365:dbl, element #10=w364:dbl, element #11=w354:dbl, element #12=w353:dbl, element #13=w352:dbl, element #14=w351:dbl, element #15=w362:dbl, element #16=w361:dbl, element #17=w360:dbl, element #18=w359:dbl, element #19=w350:dbl, element #20=w349:dbl, element #21=w348:dbl, element #22=w347:dbl)
            "L-LC-X" <- w337
            "L-LC-Y" <- w338
            "R-LC-X" <- w339
            "R-LC-Y" <- w340
            "Left Load Cell X" <- w337
            "Left Load Cell Y" <- w338
            "Right Load Cell X" <- w339
            "Right Load Cell Y" <- w340
            n102 = Add(x=w365, y=w364) -> (x+y=→"L-FP-Y":dbl)
            n103 = Add(x=w360, y=w359) -> (x+y=→"R-FP-Y":dbl)
            n104 = Add(x=w368, y=w367) -> (x+y=→"L-FP-X":dbl)
            n105 = Add(x=w362, y=w361) -> (x+y=→"R-FP-X":dbl)
            n106 = call "Center Mass (Sub VI).vi"("Z4"=w351, "Z3"=w352, "Z2"=w353, "Z1"=w354) -> ("XY Graph"=→"Center Mass Left Force Plate":cluster{dbl[], dbl[]})  [unwired: 2 in]
            n107 = call "Center Mass (Sub VI).vi"("Z4"=w347, "Z3"=w348, "Z2"=w349, "Z1"=w350) -> ("XY Graph"=w329:cluster{dbl[], dbl[]})  [unwired: 2 in]
            n108 = call "XY Graph (SubVI).vi"("Y"=w338, "X"=w337) -> ("XY Graph"=→"Left Load Cell":cluster{"array":dbl[], "array":dbl[]})
            n109 = call "XY Graph (SubVI).vi"("Y"=w340, "X"=w339) -> ("XY Graph"=→"Right Load Cell":cluster{"array":dbl[], "array":dbl[]})
            n110 = Compound Arithmetic op=ADD(w354, w353, w352, w351) -> (→"L-FP-Z" →"Left Force Plate Z" →"Left Force Plate Z":dbl)
            n111 = Compound Arithmetic op=ADD(w350, w349, w348, w347) -> (→"R-FP-Z" →"Right Force PLate Z" →"Right Force Plate Z":dbl)
            n112 = case shown="True" "?" {
              tunnel: [w395 w396] -> w330
              tunnel: w329 -> [w395 w401]
              frame False {
              }
              frame True {
                n113 = Unbundle(w401) -> (w400:dbl[], w399:dbl[])
                n114 = Multiply(x=w400, y=-1) -> (x*y=w398:dbl[])
                n115 = Bundle(w399, w398) -> (w396:cluster{dbl[], dbl[]})  [unwired: 1 in]
              }
            }
            "Center Mass Right Force Plate" <- w330
          }
          frame #4 {
          }
          frame #5 {
            n116 = call <vilib>:"DAQmx Stop Task.vi"("task/channels in"=w418) -> ("task out"=w417:refnum<k21>)  [unwired: 13 in, 1 out]
            n117 = case shown="True" "stop" {
              tunnel: [w425 State."Stop" ("(Value Not Used)")] -> w424
              tunnel: w422 -> [w425 _]
              frame False {
              }
              frame True {
              }
            }
            n118 = call <vilib>:"DAQmx Stop Task.vi"("task/channels in"=w415) -> ("task out"=w416:refnum<k21>)  [unwired: 13 in, 1 out]
            n119 = call <vilib>:"DAQmx Clear Task.vi"("task in"=w417) -> ()  [unwired: 14 in, 1 out]
            n120 = call <vilib>:"DAQmx Clear Task.vi"("task in"=w416) -> ()  [unwired: 14 in, 1 out]
          }
        }
      }
      frame "Stop" {
        n121 = Two Button Dialog(message="Do you want to stop the program?") -> (T button?=w434:bool)  [unwired: 2 in]
        n122 = case shown="False" w434 {
          tunnel: [FALSE w444] -> w432
          tunnel: [State."Main" ("(Value Not Used)") w445] -> w433
          tunnel: w431 -> [w436 w443]
          tunnel: [w437 w446] -> w430
          frame False {
            n123 = property on="stop" class="Bool (strict)"(error in=w436, "Value"=FALSE ("stop")) -> (error out=w437:errorcluster)  [unwired: 1 in, 1 out]
          }
          frame True {
            n124 = property on="Save" class="Bool (strict)"(error in=w443) -> (error out=w442:errorcluster, "Value"=w441:bool)  [unwired: 1 in, 1 out]
            n125 = case shown="False" w441 {
              tunnel: w442 -> [w447 w454]
              tunnel: [w447 w451] -> w446
              tunnel: [State."Stop" ("(Value Not Used)") State."Stop" ("(Value Not Used)")] -> w445
              tunnel: [TRUE TRUE] -> w444
              frame False {
              }
              frame True {
                (unwired) 0 ("pos offset (0)")
                n126 = local read "Baseline Out"() -> (w464:dbl[])
                n127 = local read "refnum out"() -> (w450:refnum<file>)
                n128 = Array To Spreadsheet String(delimiter (Tab)=", ", array=w464, 3:"%.3f") -> (spreadsheet string=w452:string)
                n129 = Build Array("", "BASELINE VALUES", "LX, LY, LZ, RX, RY, RZ, LF X12, LF X34, LF Y14, LF Y23, LF Z1, LF Z2, LF Z3, LF Z4, RF X12, RF X34, RF Y14, RF Y23, RF Z1, RF Z2, RF Z3, RF Z4", w452) -> (w455:string[])
                n130 = Set File Position(offset (in bytes) (0)=0 ("pos offset (0)"), refnum=w450, from (0:start)=enum16{"start", "end", "current"}."end" ("pos mode (0:2)"), error in=w454) -> (refnum out=w459:refnum<file>, error out=w460:errorcluster)
                n131 = Write to Text File(file (use dialog)=w459, text=w455, error in=w460) -> (refnum out=w456:refnum<file>, error out=w461:errorcluster)  [unwired: 1 in, 1 out]
                n132 = Close File(refnum=w456, error in=w461) -> (error out=w451:errorcluster)  [unwired: 1 out]
              }
            }
          }
        }
      }
    }
  }
  n133 = call <vilib>:"General Error Handler.vi"("error in (no error)"=w3, "[exception action] (none:0)"=w1, "[exception code]"=43) -> ()  [unwired: 8 in, 5 out]
